vi "Read CSV Files.vi"(8 "error in (no error)":errorcluster, 11 "Series file name":string) -> (0 "error out":errorcluster, 3 "Series":u16[](array[numeric]))   [LabVIEW 2018]
uses:
  <vilib>/Utility/file.llb/Read Delimited Spreadsheet (I64).vi
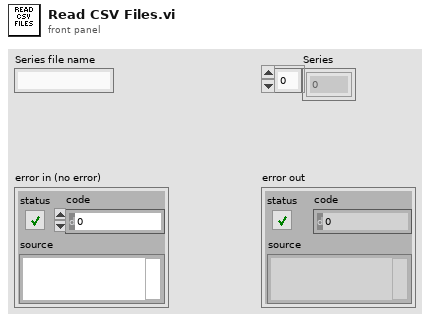
[diagram p1: front panel]
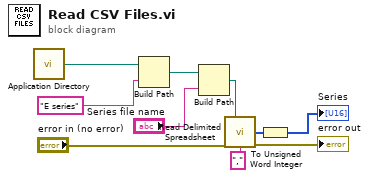
[diagram p0: block diagram]
diagram:
  n1 = call <vilib>:"Application Directory.vi"() -> ("Application Directory"=w9:path)
  n2 = Build Path(base path=w9, name or relative path="E series") -> (appended path=w7:path)
  n3 = Build Path(base path=w7, name or relative path="Series file name") -> (appended path=w5:path)
  n4 = call-poly <vilib>:"Read Delimited Spreadsheet.vi"("file path (dialog if empty)"=w5, "error in (no error)"="error in (no error)", "delimiter (\\t)"="," ("delimiter (\\t)")) -> ("first row"=w2:i64[], "error out"=→"error out":errorcluster)  [unwired: 7 in, 4 out]
  n5 = To Unsigned Word Integer(number=w2) -> (unsigned 16bit integer=→"Series":u16[])
